vi "LoadConf.vi"(8 "error in":errorcluster, 10 "MEC":string, 11 "QuickSilver in":refnum<class "QuickSilver.lvclass">) -> (0 "error out":errorcluster, 3 "QuickSilver out":refnum<class "QuickSilver.lvclass">)   [LabVIEW 2018, in "QuickSilver.lvclass"]
uses:
  QuickSilver.lvclass
  QuickSilver.lvclass/QuickSilver.ctl
  Global Coude.vi
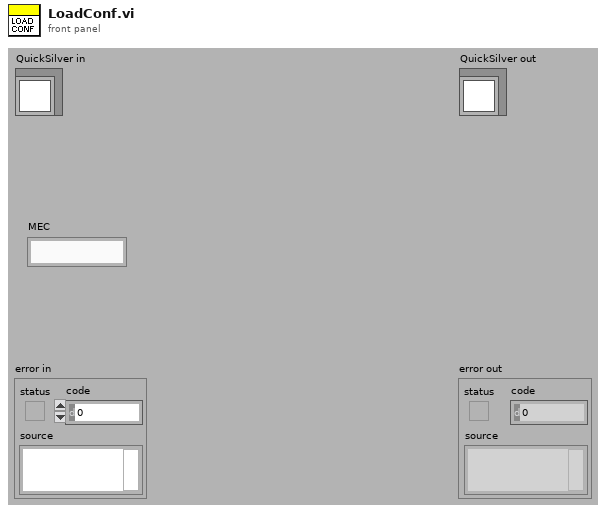
[diagram p1: front panel]
types:
  T1 = cluster{"Mec ID":string, "VISA Mec":refnum<visa-resource-name>, "Mec PosLimit":string, "Mec NegLimit":string, "Mec Factor":dbl, "Mec Speed":dbl, "Mec Acceleration":dbl, "MecOffset":string, "MecTargets":dbl[], "MecEnabled":bool, "Mec Target":dbl}
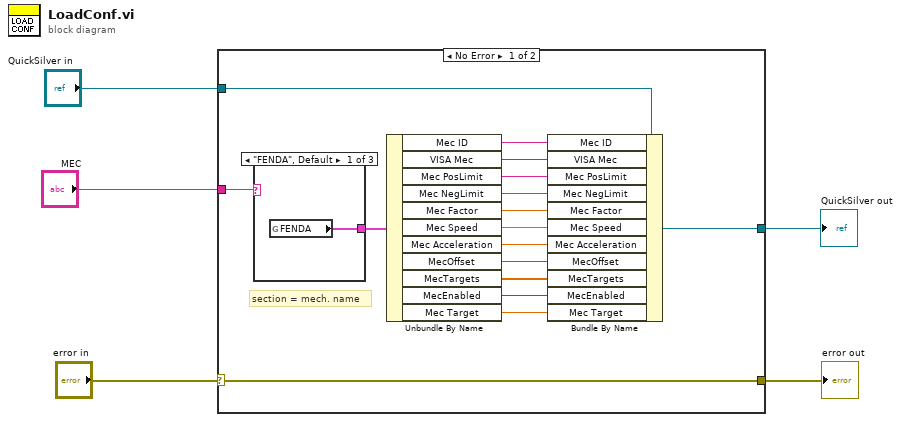
[diagram p0: block diagram]
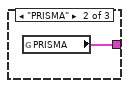
[diagram p2: hidden frame]
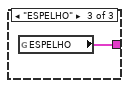
[diagram p3: hidden frame]
diagram:
  n1 = case shown="No Error" "error in" {
    selector: "error in" -> [w6 w26]
    tunnel: [w6 w26] -> w1
    tunnel: [w21 w25] -> w2
    tunnel: "QuickSilver in" -> [w20 w25]
    tunnel: "MEC" -> [w7 _]
    frame No Error {
      # "section = mech. name"
      n2 = case shown="\"FENDA\", Default" w7 {
        tunnel: [w22 w23 w24] -> w19
        frame "FENDA", Default {
          n3 = global read "Global Coude.vi" "FENDA"() -> (w22:T1)
        }
        frame "PRISMA" {
          n4 = global read "Global Coude.vi" "PRISMA"() -> (w23:T1)
        }
        frame "ESPELHO" {
          n5 = global read "Global Coude.vi" "ESPELHO"() -> (w24:T1)
        }
      }
      n6 = Unbundle By Name(w19) -> ("Mec ID"=w18:string, "VISA Mec"=w17:refnum<visa-resource-name>, "Mec PosLimit"=w16:string, "Mec NegLimit"=w15:string, "Mec Factor"=w14:dbl, "Mec Speed"=w13:dbl, "Mec Acceleration"=w12:dbl, "MecOffset"=w11:string, "MecTargets"=w10:dbl[], "MecEnabled"=w9:bool, "Mec Target"=w8:dbl)
      n7 = Bundle By Name(cluster=w20, "Mec ID"=w18, "VISA Mec"=w17, "Mec PosLimit"=w16, "Mec NegLimit"=w15, "Mec Factor"=w14, "Mec Speed"=w13, "Mec Acceleration"=w12, "MecOffset"=w11, "MecTargets"=w10, "MecEnabled"=w9, "Mec Target"=w8) -> (w21:refnum<class "QuickSilver.lvclass">)
    }
    frame Error {
    }
  }
  "error out" <- w1
  "QuickSilver out" <- w2
